vi "BRig_RT_panel_ExpStruct_v0,96.vi"(7 "input_setValues":bool, 11 "input_dataExp":u16[](array[numeric])) -> (3 "output_dataExp":u16[](array[numeric]))   [LabVIEW 2014]
panel:
  in  "ClosedLoop_LaserHold_l2":bool
  in  "ClosedLoop_LaserHold_l1":bool
  in  "FreeReward_Count2":u16
  in  "FreeReward_Count1":u16
  in  "FreeReward_Switch":bool
  in  "T_CuePenalty":u16=1000 caption="Penalty" min=1 max=10000 step=1
  in  "T_ENLPenalty":u16=100 caption="Penalty" min=10 max=10000 step=10
  in  "LaserSwitch_Probability_L1":u16
  in  "LaserSwitch":u16(slide) max=3 step=1 scale=0.0..3.0
  in  "I_allReward":bool caption="NonSpecific Lick Direction"
  in  "Tcycle_Reward_max_R":u16=1000 caption="Max" min=5 max=5000 step=5
  in  "Tcycle_Reward_min_R":u16=1000 caption="Min" min=5 max=5000 step=5
  in  "Tcycle_Reward_step_R":u16=1000 caption="Penalty" min=1 max=10000 step=1
  in  "Tcycle_Reward_max_L":u16=1000 caption="Max" min=5 max=5000 step=5
  in  "Tcycle_Reward_min_L":u16=1000 caption="Min" min=5 max=5000 step=5
  in  "Tcycle_Reward_step_L":u16=1000 caption="Penalty" min=1 max=10000 step=1
  in  "T_Cue_LED_max":u16=1000 caption="Max" min=5 max=5000 step=5
  in  "T_Cue_LED_min":u16=1000 caption="Min" min=5 max=5000 step=5
  in  "T_Cue_LED_step":u16=1000 caption="Penalty" min=1 max=10000 step=1
  in  "SolenoidProbability_L":u16=100 caption="Reward Time [ms]" min=1 max=1000 step=1
  in  "SolenoidProbability_R":u16=100 caption="Reward Time [ms]" min=1 max=1000 step=1
  in  "T_Cue_Audio_max":u16=1000 caption="Max" min=5 max=5000 step=5
  in  "T_Cue_Audio_min":u16=1000 caption="Min" min=5 max=5000 step=5
  in  "BUR_max":u16 caption="Count Reward Structure  (0 = off)"
  in  "Tcycle_Timeout":u16=1000 caption="Timeout Time [ms]" min=10 max=10000 step=1
  in  "Tcycle_Wrong":u16=1000 caption="Wrong Time [ms]" min=10 max=10000 step=1
  in  "Tcycle_Selection":u16=1000 caption="Answer Time [ms]" min=1 max=10000 step=1
  in  "Tcycle_RewardPost":u16=1000 caption="Consumption Time [ms]" min=250 max=10000 step=250
  in  "TpB_Max_R":u16=4 caption="Max TrialsPerBlock" min=1 max=12 step=1
  in  "TpB_Min_R":u16=4 caption="Min TrialsPerBlock" min=1 max=12 step=1
  in  "TpB_Max_L":u16=4 caption="Max TrialsPerBlock" min=1 max=12 step=1
  in  "TpB_Min_L":u16=4 caption="Min TrialsPerBlock" min=1 max=12 step=1
  in  "BUR_min":u16 caption="Count Reward Structure\n(0 = off)"
  in  "TrialUntilReward":bool caption="Ignore Wrong Selection"
  in  "T_Cue_Audio_step":u16=1000 caption="Penalty" min=1 max=10000 step=1
  in  "T_ENL_step":u16=100 caption="Penalty" min=10 max=10000 step=10
  in  "T_ENL_max":u16=1000 caption="Max" min=250 max=10000 step=250
  in  "T_ENL_min":u16=1000 caption="Min" min=250 max=10000 step=250
  # "Experiment Task Structure"
  # "(Laser1 or Laser2)\nLaser1 probability"
  # "Min            Max               Step        Penalty"
  # "Enforced\nNonLick"
  # "(ClosedLoop Structure)"
  # "Hold Laser1"
  # "Hold Laser2"
  # "Cue Audio"
  # "Cue LED"
  # "Selection"
  # "Reward - Dispense Water"
  # "Min            Max            StepSize"
  # "Left"
  # "Right"
  # "Dispense Water Probability"
  # "%"
  # "Left"
  # "Min"
  # "Max"
  # "Right"
  # "%"
  # "Trial Per Block Structure \n               Left                        Right"
  # "Reward - Consumption"
  # "Min"
  # "Penalty - Wrong Choice"
  # "Max"
  # "Penalty - Choice Timeout"
  # "# consecutive ReBiasing trials"
  # "Give Reward\nIf Too Many Errors"
  # "# consecutive NonForcedError trials"
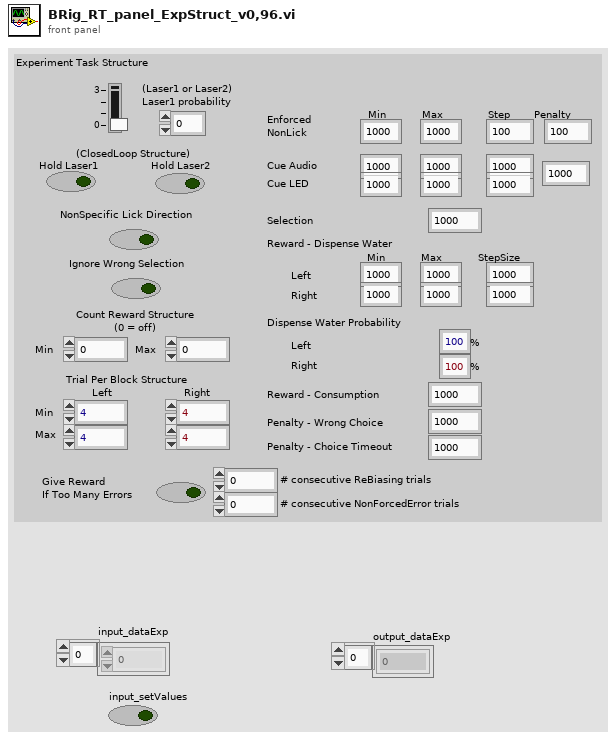
[diagram p1: front panel]
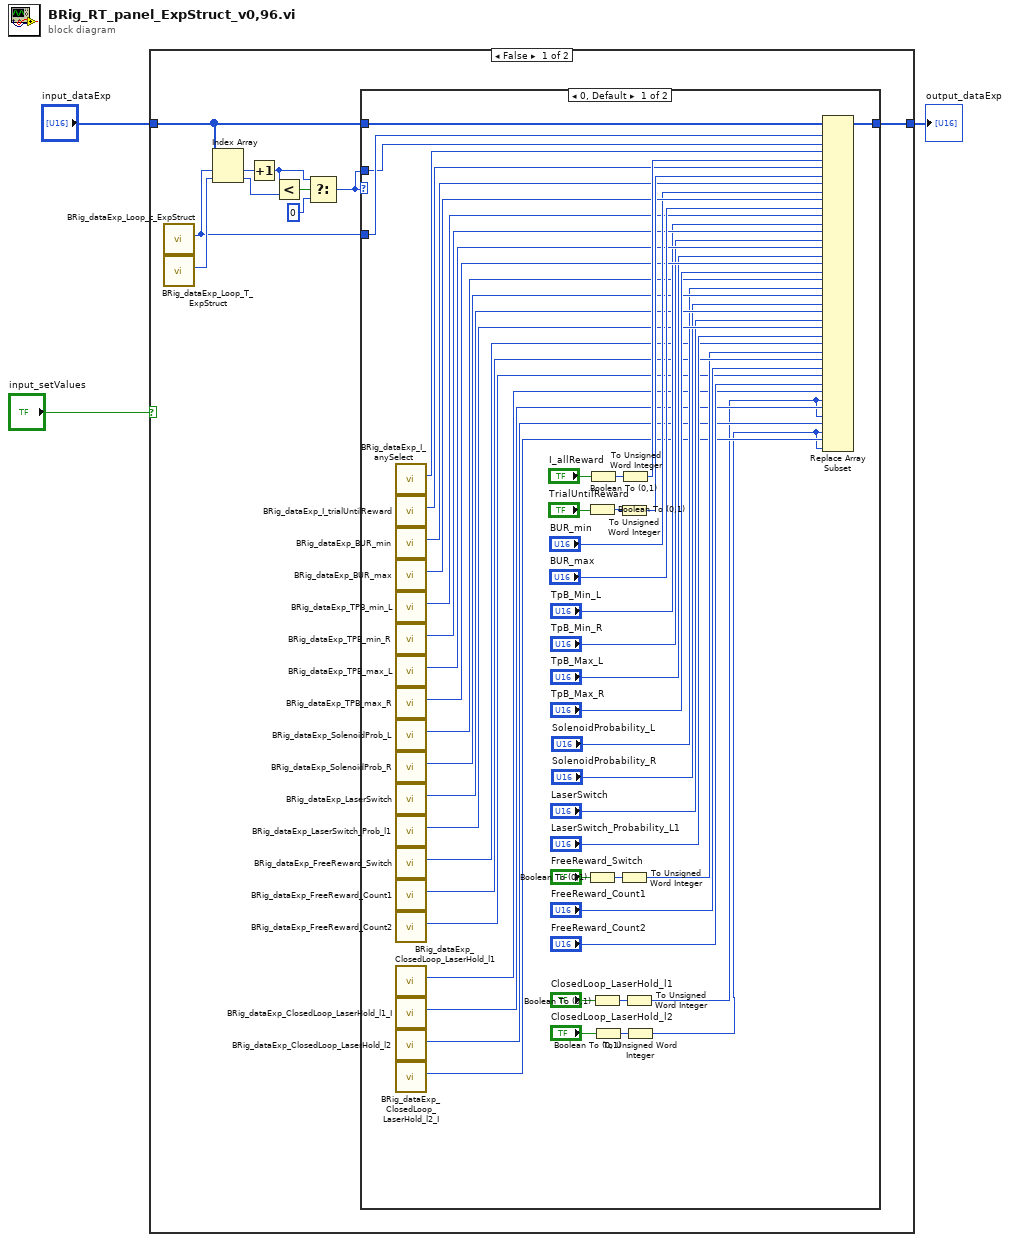
[diagram p0: block diagram]
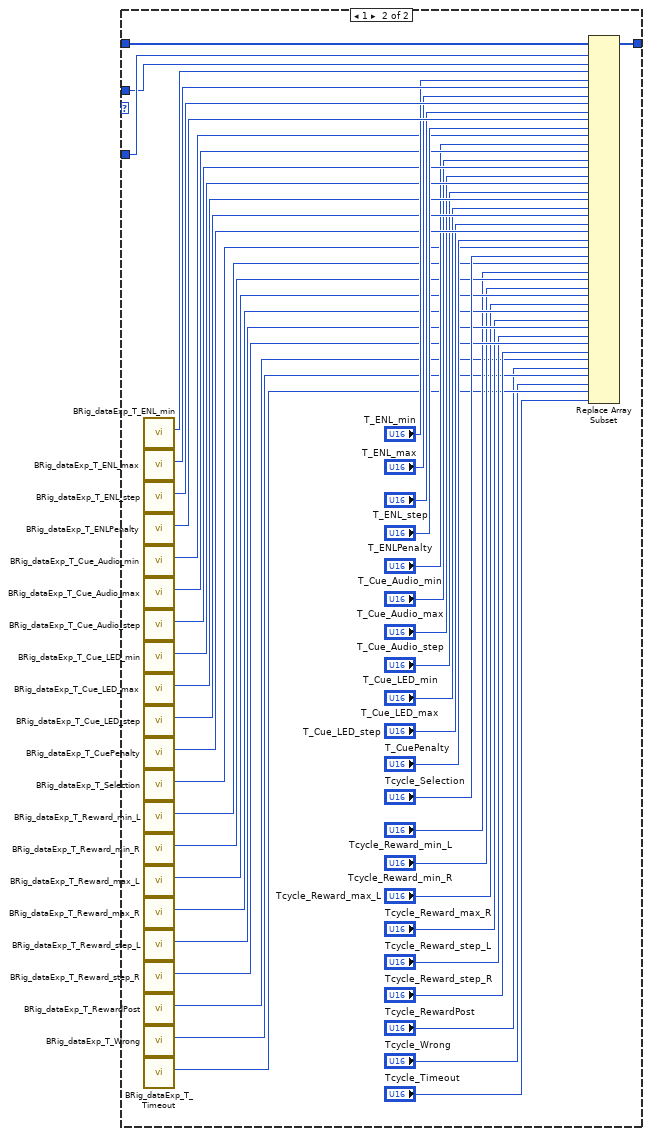
[diagram p2: hidden frame]
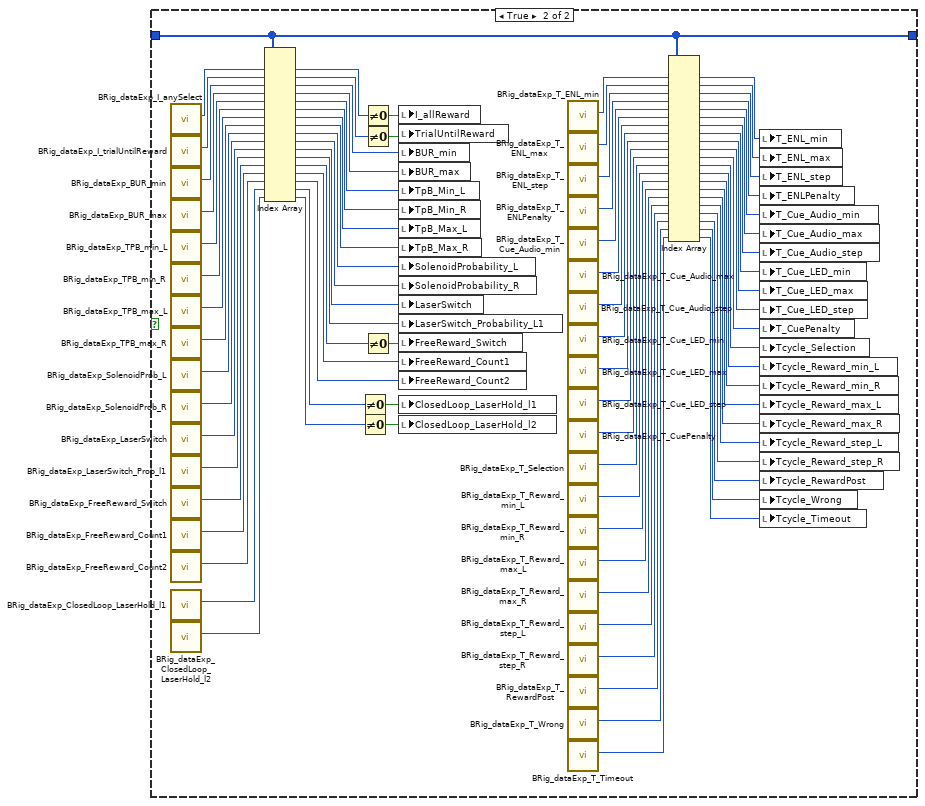
[diagram p3: hidden frame]
diagram:
  n1 = case shown="False" "input_setValues" {
    tunnel: [w13 w160] -> w3
    tunnel: "input_dataExp" -> [w12 w160]
    frame False {
      n2 = call "BRig_dataExp_Loop_c_ExpStruct.vi"() -> ("output_Loop_c_ExpStruct"=w6:i32)  [unwired: 11 in]
      n3 = call "BRig_dataExp_Loop_T_ExpStruct.vi"() -> ("output_Loop_T_ExpStruct"=w11:i32)  [unwired: 11 in]
      n4 = Index Array(array=w12, index #1=w6, index #2=w11) -> (element #1=w10:u16, element #2=w9:u16)
      n5 = Increment(x=w10) -> (x+1=w5:u16)
      n6 = Less?(x=w5, y=w9) -> (x < y?=w8:bool)
      n7 = Select(t=w5, s=w8, f=u16 0) -> (s? t:f=w4:u16)
      n8 = case shown="0, Default" w4 {
        tunnel: w12 -> [w63 w109]
        tunnel: [w62 w108] -> w13
        tunnel: w6 -> [w33 w107]
        tunnel: w4 -> [w32 w106]
        frame 0, Default {
          n9 = call "BRig_dataExp_I_anySelect.vi"() -> ("output_I_anySelect"=w61:i32)  [unwired: 11 in]
          n10 = call "BRig_dataExp_I_trialUntilReward.vi"() -> ("output_I_trialUntilReward"=w57:i32)  [unwired: 11 in]
          n11 = call "BRig_dataExp_BUR_min.vi"() -> ("output_BUR_min"=w53:i32)  [unwired: 11 in]
          n12 = call "BRig_dataExp_BUR_max.vi"() -> ("output_BUR_max"=w52:i32)  [unwired: 11 in]
          n13 = call "BRig_dataExp_TPB_min_L.vi"() -> ("output_TPB_min_L"=w49:i32)  [unwired: 11 in]
          n14 = call "BRig_dataExp_TPB_min_R.vi"() -> ("output_TPB_min_R"=w48:i32)  [unwired: 11 in]
          n15 = call "BRig_dataExp_TPB_max_L.vi"() -> ("output_TPB_max_L"=w47:i32)  [unwired: 11 in]
          n16 = call "BRig_dataExp_TPB_max_R.vi"() -> ("output_TPB_max_R"=w46:i32)  [unwired: 11 in]
          n17 = call "BRig_dataExp_SolenoidProb_L.vi"() -> ("output_SolenoidProbability_L"=w41:i32)  [unwired: 11 in]
          n18 = call "BRig_dataExp_SolenoidProb_R.vi"() -> ("output_SolenoidProbability_R"=w40:i32)  [unwired: 11 in]
          n19 = call "BRig_dataExp_LaserSwitch.vi"() -> ("output_LaserSwitch"=w39:i32)  [unwired: 11 in]
          n20 = call "BRig_dataExp_LaserSwitch_Prob_l1.vi"() -> ("output_LaserSwitch_Probability_L1"=w38:i32)  [unwired: 11 in]
          n21 = call "BRig_dataExp_FreeReward_Switch.vi"() -> ("output_FreeReward_Switch"=w29:i32)  [unwired: 11 in]
          n22 = call "BRig_dataExp_FreeReward_Count1.vi"() -> ("output_FreeReward_Count"=w28:i32)  [unwired: 11 in]
          n23 = call "BRig_dataExp_FreeReward_Count2.vi"() -> ("output_FreeReward_Count"=w25:i32)  [unwired: 11 in]
          n24 = call "BRig_dataExp_ClosedLoop_LaserHold_l1.vi"() -> ("output_CloseLoop_LaserHold_l1"=w23:i32)  [unwired: 11 in]
          n25 = call "BRig_dataExp_ClosedLoop_LaserHold_l1_I.vi"() -> ("output_CloseLoop_LaserHold_l1_I"=w22:i32)  [unwired: 11 in]
          n26 = call "BRig_dataExp_ClosedLoop_LaserHold_l2.vi"() -> ("output_CloseLoop_LaserHold_l2"=w21:i32)  [unwired: 11 in]
          n27 = call "BRig_dataExp_ClosedLoop_LaserHold_l2_I.vi"() -> ("output_CloseLoop_LaserHold_l2_I"=w20:i32)  [unwired: 11 in]
          n28 = Boolean To (0,1)(Boolean="TrialUntilReward") -> (0, 1=w56:i16)
          n29 = Boolean To (0,1)(Boolean="FreeReward_Switch") -> (0, 1=w31:i16)
          n30 = Boolean To (0,1)(Boolean="I_allReward") -> (0, 1=w59:i16)
          n31 = Boolean To (0,1)(Boolean="ClosedLoop_LaserHold_l1") -> (0, 1=w19:i16)
          n32 = Boolean To (0,1)(Boolean="ClosedLoop_LaserHold_l2") -> (0, 1=w17:i16)
          n33 = To Unsigned Word Integer(number=w56) -> (unsigned 16bit integer=w54:u16)
          n34 = To Unsigned Word Integer(number=w31) -> (unsigned 16bit integer=w27:u16)
          n35 = To Unsigned Word Integer(number=w59) -> (unsigned 16bit integer=w58:u16)
          n36 = To Unsigned Word Integer(number=w19) -> (unsigned 16bit integer=w15:u16)
          n37 = To Unsigned Word Integer(number=w17) -> (unsigned 16bit integer=w14:u16)
          n38 = Replace Array Subset(array=w63, new element #1=w32, index #1=w33, new element #2=w58, index #2=w61, new element #3=w54, index #3=w57, new element #4="BUR_min", index #4=w53, new element #5="BUR_max", index #5=w52, new element #6="TpB_Min_L", index #6=w49, new element #7="TpB_Min_R", index #7=w48, new element #8="TpB_Max_L", index #8=w47, new element #9="TpB_Max_R", index #9=w46, new element #10="SolenoidProbability_L", index #10=w41, new element #11="SolenoidProbability_R", index #11=w40, new element #12="LaserSwitch", index #12=w39, new element #13="LaserSwitch_Probability_L1", index #13=w38, new element #14=w27, index #14=w29, new element #15="FreeReward_Count1", index #15=w28, new element #16="FreeReward_Count2", index #16=w25, new element #17=w15, index #17=w23, new element #18=w15, index #18=w22, new element #19=w14, index #19=w21, new element #20=w14, index #20=w20) -> (w62:u16[])
        }
        frame 1 {
          n39 = call "BRig_dataExp_T_ENL_min.vi"() -> ("output_T_ENL_min"=w105:i32)  [unwired: 11 in]
          n40 = call "BRig_dataExp_T_ENL_max.vi"() -> ("output_T_ENL_max"=w104:i32)  [unwired: 11 in]
          n41 = call "BRig_dataExp_T_ENL_step.vi"() -> ("output_T_ENL_step"=w103:i32)  [unwired: 11 in]
          n42 = call "BRig_dataExp_T_ENLPenalty.vi"() -> ("output_ENL_penalty"=w102:i32)  [unwired: 11 in]
          n43 = call "BRig_dataExp_T_Cue_Audio_min.vi"() -> ("output_T_Cue_Audio_min"=w97:i32)  [unwired: 11 in]
          n44 = call "BRig_dataExp_T_Cue_Audio_max.vi"() -> ("output_T_Cue_Audio_max"=w96:i32)  [unwired: 11 in]
          n45 = call "BRig_dataExp_T_Cue_Audio_step.vi"() -> ("output_T_Cue_Audio_step"=w95:i32)  [unwired: 11 in]
          n46 = call "BRig_dataExp_T_Cue_LED_min.vi"() -> ("output_T_Cue_LED_min"=w94:i32)  [unwired: 11 in]
          n47 = call "BRig_dataExp_T_Cue_LED_max.vi"() -> ("output_T_Cue_LED_max"=w93:i32)  [unwired: 11 in]
          n48 = call "BRig_dataExp_T_Cue_LED_step.vi"() -> ("output_T_Cue_LED_step"=w92:i32)  [unwired: 11 in]
          n49 = call "BRig_dataExp_T_CuePenalty.vi"() -> ("output_T_CuePenalty"=w91:i32)  [unwired: 11 in]
          n50 = call "BRig_dataExp_T_Selection.vi"() -> ("output_T_Selection"=w83:i32)  [unwired: 11 in]
          n51 = call "BRig_dataExp_T_Reward_min_L.vi"() -> ("output_Tcycle_Reward_min_L"=w81:i32)  [unwired: 11 in]
          n52 = call "BRig_dataExp_T_Reward_min_R.vi"() -> ("output_T_Reward_min_R"=w80:i32)  [unwired: 11 in]
          n53 = call "BRig_dataExp_T_Reward_max_L.vi"() -> ("output_T_Reward_max_L"=w79:i32)  [unwired: 11 in]
          n54 = call "BRig_dataExp_T_Reward_max_R.vi"() -> ("output_T_Reward_max_R"=w78:i32)  [unwired: 11 in]
          n55 = call "BRig_dataExp_T_Reward_step_L.vi"() -> ("output_T_Reward_step_L"=w77:i32)  [unwired: 11 in]
          n56 = call "BRig_dataExp_T_Reward_step_R.vi"() -> ("output_T_Reward_step_R"=w76:i32)  [unwired: 11 in]
          n57 = call "BRig_dataExp_T_RewardPost.vi"() -> ("output_T_RewardPost"=w69:i32)  [unwired: 11 in]
          n58 = call "BRig_dataExp_T_Wrong.vi"() -> ("output_T_Wrong"=w68:i32)  [unwired: 11 in]
          n59 = call "BRig_dataExp_T_Timeout.vi"() -> ("output_T_Timeout"=w67:i32)  [unwired: 11 in]
          n60 = Replace Array Subset(array=w109, new element #1=w106, index #1=w107, new element #2="T_ENL_min", index #2=w105, new element #3="T_ENL_max", index #3=w104, new element #4="T_ENL_step", index #4=w103, new element #5="T_ENLPenalty", index #5=w102, new element #6="T_Cue_Audio_min", index #6=w97, new element #7="T_Cue_Audio_max", index #7=w96, new element #8="T_Cue_Audio_step", index #8=w95, new element #9="T_Cue_LED_min", index #9=w94, new element #10="T_Cue_LED_max", index #10=w93, new element #11="T_Cue_LED_step", index #11=w92, new element #12="T_CuePenalty", index #12=w91, new element #13="Tcycle_Selection", index #13=w83, new element #14="Tcycle_Reward_min_L", index #14=w81, new element #15="Tcycle_Reward_min_R", index #15=w80, new element #16="Tcycle_Reward_max_L", index #16=w79, new element #17="Tcycle_Reward_max_R", index #17=w78, new element #18="Tcycle_Reward_step_L", index #18=w77, new element #19="Tcycle_Reward_step_R", index #19=w76, new element #20="Tcycle_RewardPost", index #20=w69, new element #21="Tcycle_Wrong", index #21=w68, new element #22="Tcycle_Timeout", index #22=w67) -> (w108:u16[])
        }
      }
    }
    frame True {
      n61 = call "BRig_dataExp_I_anySelect.vi"() -> ("output_I_anySelect"=w191:i32)  [unwired: 11 in]
      n62 = call "BRig_dataExp_I_trialUntilReward.vi"() -> ("output_I_trialUntilReward"=w190:i32)  [unwired: 11 in]
      n63 = call "BRig_dataExp_BUR_min.vi"() -> ("output_BUR_min"=w189:i32)  [unwired: 11 in]
      n64 = call "BRig_dataExp_BUR_max.vi"() -> ("output_BUR_max"=w188:i32)  [unwired: 11 in]
      n65 = call "BRig_dataExp_TPB_min_L.vi"() -> ("output_TPB_min_L"=w187:i32)  [unwired: 11 in]
      n66 = call "BRig_dataExp_TPB_min_R.vi"() -> ("output_TPB_min_R"=w186:i32)  [unwired: 11 in]
      n67 = call "BRig_dataExp_TPB_max_L.vi"() -> ("output_TPB_max_L"=w185:i32)  [unwired: 11 in]
      n68 = call "BRig_dataExp_TPB_max_R.vi"() -> ("output_TPB_max_R"=w184:i32)  [unwired: 11 in]
      n69 = call "BRig_dataExp_SolenoidProb_L.vi"() -> ("output_SolenoidProbability_L"=w183:i32)  [unwired: 11 in]
      n70 = call "BRig_dataExp_SolenoidProb_R.vi"() -> ("output_SolenoidProbability_R"=w182:i32)  [unwired: 11 in]
      n71 = call "BRig_dataExp_LaserSwitch.vi"() -> ("output_LaserSwitch"=w181:i32)  [unwired: 11 in]
      n72 = call "BRig_dataExp_LaserSwitch_Prob_l1.vi"() -> ("output_LaserSwitch_Probability_L1"=w180:i32)  [unwired: 11 in]
      n73 = call "BRig_dataExp_FreeReward_Switch.vi"() -> ("output_FreeReward_Switch"=w179:i32)  [unwired: 11 in]
      n74 = call "BRig_dataExp_FreeReward_Count1.vi"() -> ("output_FreeReward_Count"=w178:i32)  [unwired: 11 in]
      n75 = call "BRig_dataExp_FreeReward_Count2.vi"() -> ("output_FreeReward_Count"=w117:i32)  [unwired: 11 in]
      n76 = call "BRig_dataExp_ClosedLoop_LaserHold_l1.vi"() -> ("output_CloseLoop_LaserHold_l1"=w115:i32)  [unwired: 11 in]
      n77 = call "BRig_dataExp_ClosedLoop_LaserHold_l2.vi"() -> ("output_CloseLoop_LaserHold_l2"=w114:i32)  [unwired: 11 in]
      n78 = Index Array(array=w160, index #1=w191, index #2=w190, index #3=w189, index #4=w188, index #5=w187, index #6=w186, index #7=w185, index #8=w184, index #9=w183, index #10=w182, index #11=w181, index #12=w180, index #13=w179, index #14=w178, index #15=w117, index #16=w115, index #17=w114) -> (element #1=w174:u16, element #2=w173:u16, element #3=w172:u16, element #4=w171:u16, element #5=w170:u16, element #6=w169:u16, element #7=w168:u16, element #8=w167:u16, element #9=w166:u16, element #10=w165:u16, element #11=w164:u16, element #12=w163:u16, element #13=w162:u16, element #14=w161:u16, element #15=w116:u16, element #16=w111:u16, element #17=w110:u16)
      n79 = Not Equal To 0?(x=w111) -> (x != 0?=w113:bool)
      n80 = Not Equal To 0?(x=w110) -> (x != 0?=w112:bool)
      n81 = Not Equal To 0?(x=w174) -> (x != 0?=w177:bool)
      n82 = Not Equal To 0?(x=w173) -> (x != 0?=w176:bool)
      n83 = Not Equal To 0?(x=w162) -> (x != 0?=w175:bool)
      n84 = local write "I_allReward"(w177) -> ()
      n85 = local write "TrialUntilReward"(w176) -> ()
      n86 = local write "BUR_min"(w172) -> ()
      n87 = local write "BUR_max"(w171) -> ()
      n88 = local write "TpB_Min_L"(w170) -> ()
      n89 = local write "TpB_Min_R"(w169) -> ()
      n90 = local write "TpB_Max_L"(w168) -> ()
      n91 = local write "TpB_Max_R"(w167) -> ()
      n92 = local write "SolenoidProbability_L"(w166) -> ()
      n93 = local write "SolenoidProbability_R"(w165) -> ()
      n94 = local write "LaserSwitch"(w164) -> ()
      n95 = local write "LaserSwitch_Probability_L1"(w163) -> ()
      n96 = local write "FreeReward_Switch"(w175) -> ()
      n97 = local write "FreeReward_Count1"(w161) -> ()
      n98 = local write "FreeReward_Count2"(w116) -> ()
      n99 = local write "ClosedLoop_LaserHold_l1"(w113) -> ()
      n100 = local write "ClosedLoop_LaserHold_l2"(w112) -> ()
      n101 = call "BRig_dataExp_T_ENL_min.vi"() -> ("output_T_ENL_min"=w159:i32)  [unwired: 11 in]
      n102 = call "BRig_dataExp_T_ENL_max.vi"() -> ("output_T_ENL_max"=w158:i32)  [unwired: 11 in]
      n103 = call "BRig_dataExp_T_ENL_step.vi"() -> ("output_T_ENL_step"=w157:i32)  [unwired: 11 in]
      n104 = call "BRig_dataExp_T_ENLPenalty.vi"() -> ("output_ENL_penalty"=w156:i32)  [unwired: 11 in]
      n105 = call "BRig_dataExp_T_Cue_Audio_min.vi"() -> ("output_T_Cue_Audio_min"=w155:i32)  [unwired: 11 in]
      n106 = call "BRig_dataExp_T_Cue_Audio_max.vi"() -> ("output_T_Cue_Audio_max"=w154:i32)  [unwired: 11 in]
      n107 = call "BRig_dataExp_T_Cue_Audio_step.vi"() -> ("output_T_Cue_Audio_step"=w153:i32)  [unwired: 11 in]
      n108 = call "BRig_dataExp_T_Cue_LED_min.vi"() -> ("output_T_Cue_LED_min"=w152:i32)  [unwired: 11 in]
      n109 = call "BRig_dataExp_T_Cue_LED_max.vi"() -> ("output_T_Cue_LED_max"=w151:i32)  [unwired: 11 in]
      n110 = call "BRig_dataExp_T_Cue_LED_step.vi"() -> ("output_T_Cue_LED_step"=w150:i32)  [unwired: 11 in]
      n111 = call "BRig_dataExp_T_CuePenalty.vi"() -> ("output_T_CuePenalty"=w149:i32)  [unwired: 11 in]
      n112 = call "BRig_dataExp_T_Selection.vi"() -> ("output_T_Selection"=w148:i32)  [unwired: 11 in]
      n113 = call "BRig_dataExp_T_Reward_min_L.vi"() -> ("output_Tcycle_Reward_min_L"=w147:i32)  [unwired: 11 in]
      n114 = call "BRig_dataExp_T_Reward_min_R.vi"() -> ("output_T_Reward_min_R"=w146:i32)  [unwired: 11 in]
      n115 = call "BRig_dataExp_T_Reward_max_L.vi"() -> ("output_T_Reward_max_L"=w145:i32)  [unwired: 11 in]
      n116 = call "BRig_dataExp_T_Reward_max_R.vi"() -> ("output_T_Reward_max_R"=w144:i32)  [unwired: 11 in]
      n117 = call "BRig_dataExp_T_Reward_step_L.vi"() -> ("output_T_Reward_step_L"=w143:i32)  [unwired: 11 in]
      n118 = call "BRig_dataExp_T_Reward_step_R.vi"() -> ("output_T_Reward_step_R"=w142:i32)  [unwired: 11 in]
      n119 = call "BRig_dataExp_T_RewardPost.vi"() -> ("output_T_RewardPost"=w141:i32)  [unwired: 11 in]
      n120 = call "BRig_dataExp_T_Wrong.vi"() -> ("output_T_Wrong"=w140:i32)  [unwired: 11 in]
      n121 = call "BRig_dataExp_T_Timeout.vi"() -> ("output_T_Timeout"=w139:i32)  [unwired: 11 in]
      n122 = Index Array(array=w160, index #1=w159, index #2=w158, index #3=w157, index #4=w156, index #5=w155, index #6=w154, index #7=w153, index #8=w152, index #9=w151, index #10=w150, index #11=w149, index #12=w148, index #13=w147, index #14=w146, index #15=w145, index #16=w144, index #17=w143, index #18=w142, index #19=w141, index #20=w140, index #21=w139) -> (element #1=w138:u16, element #2=w137:u16, element #3=w136:u16, element #4=w135:u16, element #5=w134:u16, element #6=w133:u16, element #7=w132:u16, element #8=w131:u16, element #9=w130:u16, element #10=w129:u16, element #11=w128:u16, element #12=w127:u16, element #13=w126:u16, element #14=w125:u16, element #15=w124:u16, element #16=w123:u16, element #17=w122:u16, element #18=w121:u16, element #19=w120:u16, element #20=w119:u16, element #21=w118:u16)
      n123 = local write "T_ENL_min"(w138) -> ()
      n124 = local write "T_ENL_max"(w137) -> ()
      n125 = local write "T_ENL_step"(w136) -> ()
      n126 = local write "T_ENLPenalty"(w135) -> ()
      n127 = local write "T_Cue_Audio_min"(w134) -> ()
      n128 = local write "T_Cue_Audio_max"(w133) -> ()
      n129 = local write "T_Cue_Audio_step"(w132) -> ()
      n130 = local write "T_Cue_LED_min"(w131) -> ()
      n131 = local write "T_Cue_LED_max"(w130) -> ()
      n132 = local write "T_Cue_LED_step"(w129) -> ()
      n133 = local write "T_CuePenalty"(w128) -> ()
      n134 = local write "Tcycle_Selection"(w127) -> ()
      n135 = local write "Tcycle_Reward_min_L"(w126) -> ()
      n136 = local write "Tcycle_Reward_min_R"(w125) -> ()
      n137 = local write "Tcycle_Reward_max_L"(w124) -> ()
      n138 = local write "Tcycle_Reward_max_R"(w123) -> ()
      n139 = local write "Tcycle_Reward_step_L"(w122) -> ()
      n140 = local write "Tcycle_Reward_step_R"(w121) -> ()
      n141 = local write "Tcycle_RewardPost"(w120) -> ()
      n142 = local write "Tcycle_Wrong"(w119) -> ()
      n143 = local write "Tcycle_Timeout"(w118) -> ()
    }
  }
  "output_dataExp" <- w3
